vi "AO Python Write TCP Data.vi"(0 "Connection ID":refnum<k5>, 7 "Write String":string, 11 "Error":errorcluster, 13 "Timeout (ms)":i32=5000) -> (4 "Connection ID (Dup)":refnum<k5>, 15 "Error Out":errorcluster)   [LabVIEW 2016]
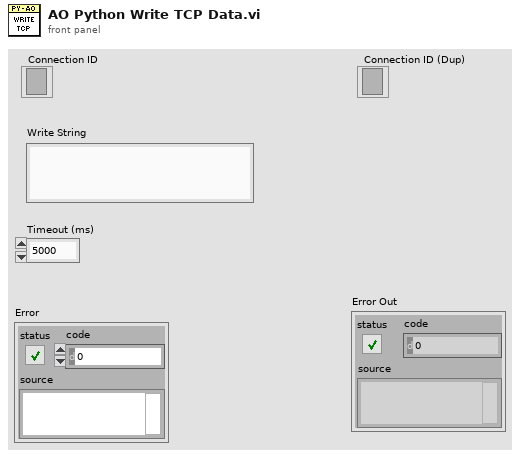
[diagram p1: front panel]
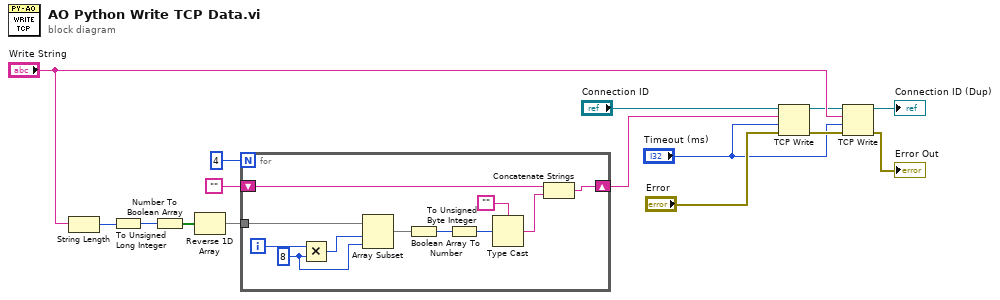
[diagram p0: block diagram]
diagram:
  n1 = String Length(string="Write String") -> (length=w15:i32)
  n2 = To Unsigned Long Integer(number=w15) -> (unsigned 32bit integer=w14:u32)
  n3 = Number To Boolean Array(number=w14) -> (Boolean array=w12:bool[])
  n4 = Reverse 1D Array(array=w12) -> (reversed array=w10:bool[])
  n5 = for {
    N: 4 -> [_]
    tunnel: w10 -> [w26]
    shift-right: [w19] -> w9
    shift-left: "" -> [w20]
    i -> [w25]
    w23 = 8 ("y")
    n6 = Multiply(x=w25, y=w23) -> (x*y=w24:i32)
    n7 = Array Subset(array=w26, index=w24, length=w23) -> (w22:bool[])
    n8 = Boolean Array To Number(Boolean array=w22) -> (number=w17:u32)
    n9 = To Unsigned Byte Integer(number=w17) -> (unsigned 8bit integer=w16:u8)
    n10 = Type Cast(type="", x=w16) -> (*(type *) &x=w18:string)
    n11 = Concatenate Strings(w20, w18) -> (w19:string)
  }
  n12 = TCP Write(connection ID="Connection ID", data in=w9, error in (no error)="Error", 9:"Timeout (ms)") -> (connection ID out=w5:refnum<k5>, error out=w4:errorcluster)  [unwired: 1 out]
  n13 = TCP Write(connection ID=w5, data in="Write String", error in (no error)=w4, 9:"Timeout (ms)") -> (connection ID out=→"Connection ID (Dup)":refnum<k5>, error out=→"Error Out":errorcluster)  [unwired: 1 out]
